vi "3.5-Limbic.vi"() -> ()   [LabVIEW 2010]
uses:
  3.0-Global.vi
panel:
  out "Heartbeat":bool
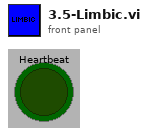
[diagram p1: front panel]
types:
  T1 = typedef "3.3-What Sensor Typedef.ctl" = cluster{"LIDAR Data":T2}
  T2 = typedef "3.3.1-LIDAR Data Typedef.ctl" = cluster{"Angle array":dbl[], "Magnitude array ":dbl[]}
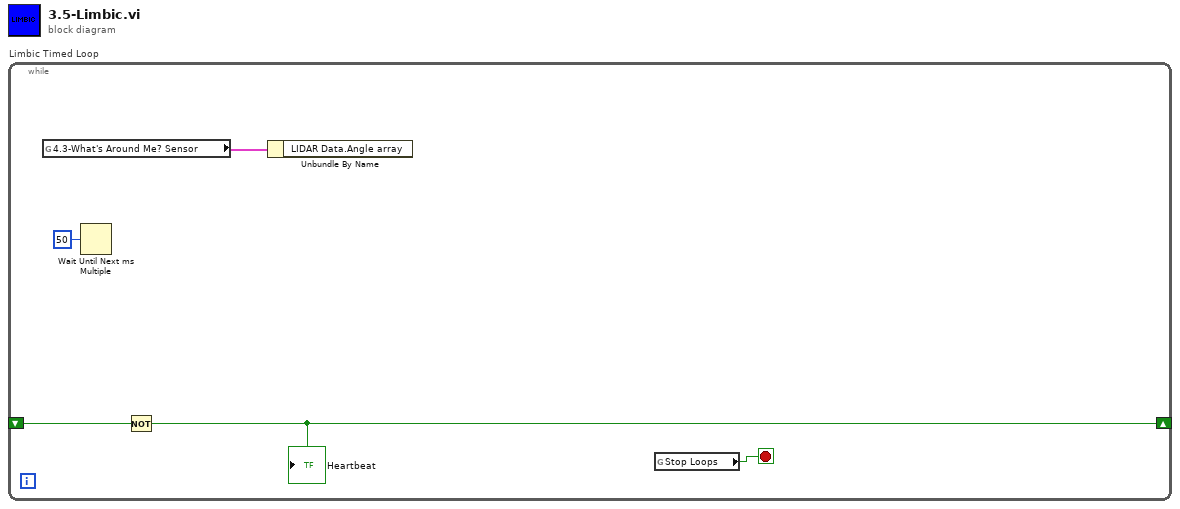
[diagram p0: block diagram]
diagram:
  n1 = while "Limbic Timed Loop" {
    shift-right: [w4] -> _
    shift-left: _ -> [w5]
    stop <- w3 stop-if-true
    n2 = global read "3.0-Global.vi" "4.3-What's Around Me? Sensor"() -> (w2:T1)
    n3 = Wait Until Next ms Multiple(millisecond multiple=u32 50) -> ()  [unwired: 1 out]
    n4 = Not(x=w5) -> (.not. x?=w4:bool)
    "Heartbeat" <- w4
    n5 = Unbundle By Name(w2) -> ()  [unwired: 1 out]
    n6 = global read "3.0-Global.vi" "Stop Loops"() -> (w3:bool)
  }
